vi "Populate Attr Priv.vi"(5 "Attribute IDs":string[](array[string]), 6 "Item Indent":i32, 7 "Data Types Dict":variant, 8 "error in":errorcluster, 9 "Attribute Values":variant[](array[variant]), 10 "Attribute Names":string[](array[string]), 11 "Unique ID":string) -> (0 "error out":errorcluster, 1 "Attr Items":T1(array[cluster]))   [LabVIEW 2017, in "Tree API.lvlib" / "Tree.lvclass"]
uses:
  Tree.lvclass
  Tree Data/Tree Data.lvclass
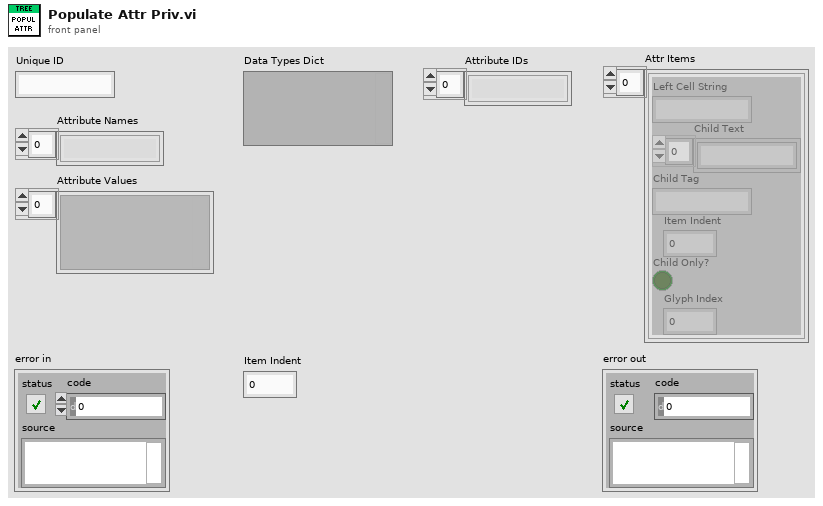
[diagram p1: front panel]
types:
  T1 = cluster{"Left Cell String":string, "Child Text":string[], "Child Tag":string, "Item Indent":i32, "Child Only?":bool, "Glyph Index":i32}[]
  T2 = cluster{"Left Cell String":string, "Child Text":string[], "Child Tag":string, "Item Indent":i32, "Child Only?":bool, "Glyph Index":i32}
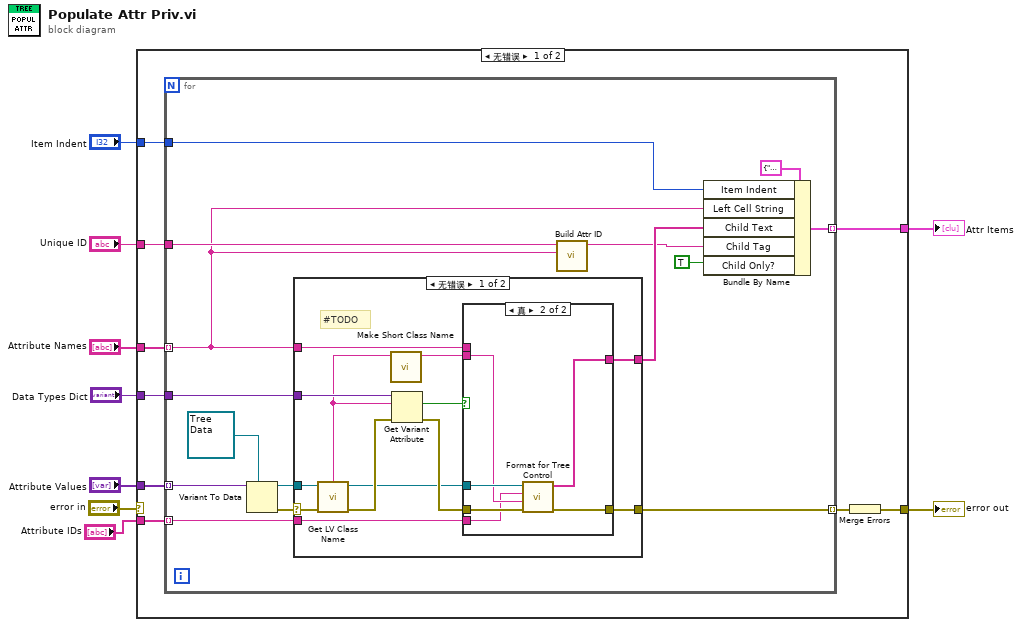
[diagram p0: block diagram]
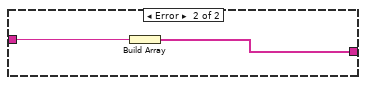
[diagram p3: hidden frame]
diagram:
  n1 = case shown="无错误" "error in" {
    selector: "error in" -> [_ w55]
    tunnel: "Unique ID" -> [w18 _]
    tunnel: "Attribute Names" -> [w17 _]
    tunnel: "Attribute Values" -> [w16 _]
    tunnel: "Data Types Dict" -> [w15 _]
    tunnel: [w13 w55] -> w5
    tunnel: "Item Indent" -> [w12 _]
    tunnel: [w11 _] -> w2
    tunnel: "Attribute IDs" -> [w10 _]
    frame No Error {
      n2 = for {
        tunnel: w17 -> [w20] mode=indexing
        tunnel: w18 -> [w23]
        tunnel: w16 -> [w33] mode=indexing
        tunnel: w15 -> [w30]
        tunnel: [w28] -> w14 mode=indexing
        tunnel: w12 -> [w22]
        tunnel: [w21] -> w11 mode=indexing
        tunnel: w10 -> [w19] mode=indexing
        n3 = Variant To Data(type=refnum<class "Tree Data.lvclass"> refnum ("Tree Data.lvclass"), Variant=w33) -> (data=w32:refnum<class "Tree Data.lvclass">, error out=w31:errorcluster)  [unwired: 1 in]
        n4 = case shown="无错误" w31 {
          selector: w31 -> [w45 _]
          tunnel: w32 -> [w40 _]
          tunnel: [w38 w53] -> w25
          tunnel: w20 -> [w39 w54]
          tunnel: w30 -> [w44 _]
          tunnel: [w37 _] -> w28
          tunnel: w19 -> [w34 _]
          frame No Error {
            # "#TODO"
            n5 = call <vilib>:"Get LV Class Name.vi"("error in (no error)"=w45, "object"=w40) -> ("error out"=w43:errorcluster, "class name"=w35:string)  [unwired: 8 in]
            n6 = call "Make Short Class Name.vi"("Class Name"=w35) -> ("Shortened Class Name"=w36:string)  [unwired: 10 in]
            n7 = Get Variant Attribute(Variant=w44, name=w35, error in=w43) -> (found=w41:bool, error out=w42:errorcluster)  [unwired: 1 in, 2 out]
            n8 = case shown="真" w41 {
              tunnel: w42 -> [w46 w51]
              tunnel: w40 -> [_ w52]
              tunnel: w39 -> [_ _]
              tunnel: w36 -> [_ w50]
              tunnel: [_ w48] -> w38
              tunnel: [w46 w49] -> w37
              tunnel: w34 -> [_ w47]
              frame False {
              }
              frame True {
                n9 = call-dynamic "Format for Tree Control.vi"("Error In"=w51, "Class Name"=w50, "Attr ID"=w47, "Tree Data"=w52) -> ("Error Out"=w49:errorcluster, "Child Text"=w48:string[])  [unwired: 6 in]
              }
            }
          }
          frame Error {
            n10 = Build Array(w54) -> (w53:string[])
          }
        }
        n11 = call "Build Attr ID.vi"("Attr Name"=w20, "Unique ID"=w23) -> ("Attr ID Out"=w24:string)  [unwired: 9 in]
        n12 = Bundle By Name(cluster=T2 {"Left Cell String"="", "Child Text"=[], "Child Tag"="", "Item Indent"=0, "Child Only?"=FALSE, "Glyph Index"=0} ("Item"), "Item Indent"=w22, "Left Cell String"=w20, "Child Text"=w25, "Child Tag"=w24, "Child Only?"=TRUE) -> (w21:T2)
      }
      n13 = Merge Errors(w14) -> (w13:errorcluster)
    }
    frame Error {
    }
  }
  "error out" <- w5
  "Attr Items" <- w2
